vi "open_rga_interface.vi"() -> ()   [LabVIEW 2016]
panel:
  in  "error in (no error)":errorcluster
  out "error out":errorcluster
  out "standard output":string
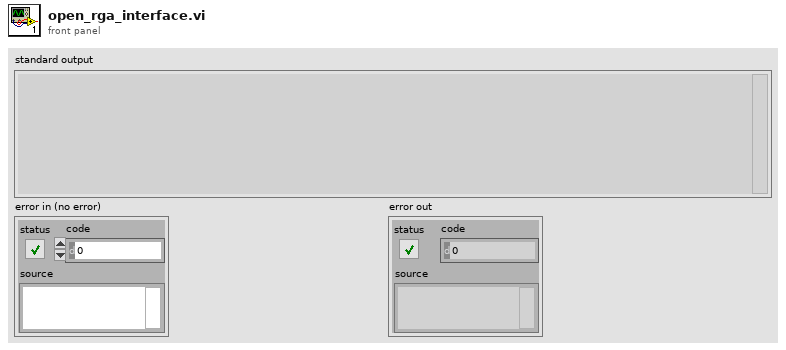
[diagram p1: front panel]
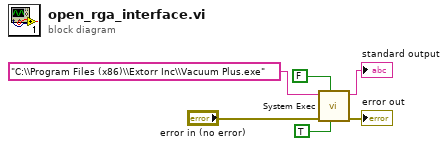
[diagram p0: block diagram]
diagram:
  n1 = call <vilib>:"System Exec.vi"("run minimized? (F)"=TRUE, "wait until completion? (T)"=FALSE, "error in (no error)"="error in (no error)", "command line"="C:\\Program Files (x86)\\Extorr Inc\\Vacuum Plus.exe") -> ("error out"=→"error out":errorcluster, "standard output"=→"standard output":string)  [unwired: 4 in, 2 out]
